vi "Read Batch Profiles(for High-Speed Mode).vi"(8 "error in (no error)":errorcluster, 9 "Data Size (0: Auto Size)":u32, 10 "Read Req":T2={"Read Area"=TRUE, "Batch Pos"=0, "Read Batch No"=0, "Read Profile No."=0, "Read Profile Cnt"=0, "Erase"=FALSE} {"Batch Pos" items=["CURRENT"=0, "SPECIFY"=2, "COMMITED"=3, "NEWEST PROFILE"=4]}, 11 "Device ID (0)":i32) -> (0 "error out":errorcluster, 1 "Profile Rsp":T1, 2 "Profile Data":u32[](array[numeric]), 3 "Device ID out":i32, 5 "Profile Info":T4={"Profile Cnt"=1, "Envelope"=FALSE, " Profile Data Point"=0, " X Start"=0, " X Pitch"=0})   [LabVIEW 2014, in "Keyence LJ-V7000.lvlib"]
doc: "This function gets profile data.\nProfile data is stored in 0.01 μm units.\n\n<B>Note</B>:\nFor the details on the data stored in the profile data (storage order and size), refer to <B>10.3</B> in a manual of measuring instrument drivers.\n\nIf Compression(timse axis) is ON, use <B>Read Profiles(for High-Speed Mode)</B> VI.\n\nTo read all of the profiles in one batch, read them with the procedure below.\n1. Call this VI by specifying <B>Current</B> for <B>Batch Pos</B> in <B>Read Req</B>. Save the start position and the amount of profiles that were read and the batch number that was read.\n2. Configure <B>Read Req</B> as listed below and call this VI again.\n　・<B>Batch Pos</B> = SPECIFY\n　・<B>Read Batch No</B> = batch number that was read\n　・<B>Read Profile Cnt</B> = starting profile number of the unread profiles in the batch\n3. Update <B>Read Profile Cnt</B> in step 2 and call this VI until all of the profiles in the batch can be read."
uses:
  Keyence LJ-V7000.lvlib
  Clusters/Profile Info.ctl
  Clusters/Read Batch Profile Req.ctl
  constant/Batch Pos.ctl
  Clusters/Read Batch Profile Rsp.ctl
  constant/Driver VI No.ctl
  Private/vi/Low Level/Make DLL Param(Read Batch Profile Req).vi
  Private/vi/Low Level/Make DLL Param(Read Batch Profile Rsp).vi
  Private/vi/Low Level/Make VI Param(Read Batch Profile Rsp).vi
panel:
  # "(c) 2012 KEYENCE CORPORATION.  ALL RIGHTS RESERVED."
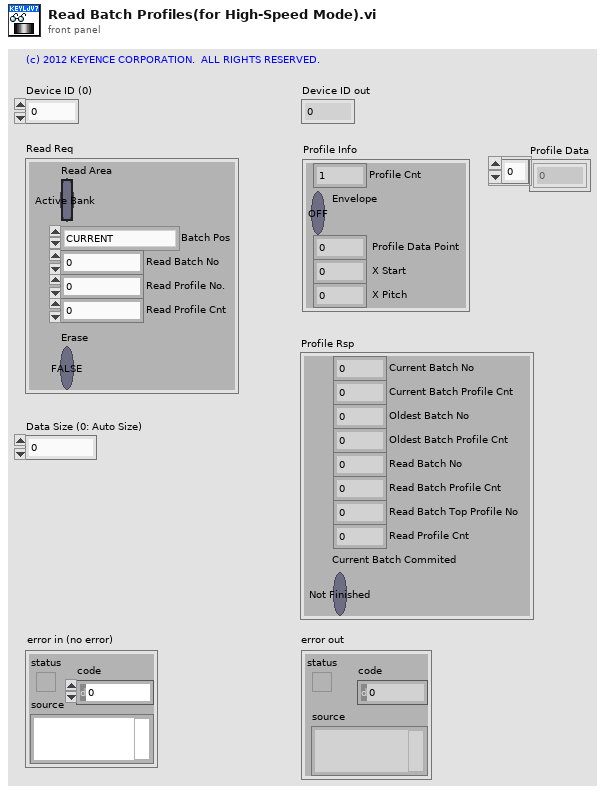
[diagram p1: front panel]
types:
  T1 = typedef "Keyence LJ-V7000.lvlib/Read Batch Profile Rsp.ctl" = cluster{"Current Batch No":u32, "Current Batch Profile Cnt":u32, "Oldest Batch No":u32, "Oldest Batch Profile Cnt":u32, "Read Batch No":u32, "Read Batch Profile Cnt":u32, "Read Batch Top Profile No":u32, "Read Profile Cnt":u8, "Current Batch Commited":bool}
  T2 = typedef "Keyence LJ-V7000.lvlib/Read Batch Profile Req.ctl" = cluster{"Read Area":bool, "Batch Pos":T3, "Read Batch No":u32, "Read Profile No.":u32, "Read Profile Cnt":u8, "Erase":bool}
  T3 = typedef "Keyence LJ-V7000.lvlib/Batch Pos.ctl" = u8
  T4 = typedef "Keyence LJ-V7000.lvlib/Profile Info.ctl" = cluster{"Profile Cnt":u8, "Envelope":bool, " Profile Data Point":u16, " X Start":i32, " X Pitch":i32}
  T5 = typedef "Keyence LJ-V7000.lvlib/Driver VI No.ctl" = enum16{"Initialize", "Close", "Reboot Controller", "Return to Factory State", "Get System Error", "Clear System Error", "Trigger", "Start Batch Measurements", "Stop Batch Measurements", "Auto Zero", "Timing", "Reset", "Clear Memory", "Set Setting", "Get Setting", "Initialize Setting", "Reflect Setting", "Update Write Settings Area", "Check Status of Saving to Save Area", "Set Time", "Get Time", "Change Program", "Read Active Program Number", "Read Measurement Data", "Read Profiles(for High-Speed Mode)", "Read Batch Profiles(for High-Speed Mode)", "Read Profiles(for Advanced Mode)", "Read Batch Profiles(for Advanced Mode)", "Start Storage", "Stop Storage", "Read Storage Status", "Read Data Storage Data", "Read Profile Storage Data", "Read Batch Profile Storage Data", "Start High-Speed Data Communication", "Stop High-Speed Data Communication", "Read Profiles(for High-Speed Communication)"}
  T6 = cluster{u8, "Batch Pos":T3, "reserve":u8, "reserve":u8, "Read Batch No":u32, "Read Profile No.":u32, "Read Profile Cnt":u8, u8, "reserve":u8, "reserve":u8}
  T7 = cluster{"Current Batch No":u32, "Current Batch Profile Cnt":u32, "Oldest Batch No":u32, "Oldest Batch Profile Cnt":u32, "Read Batch No":u32, "Read Batch Profile Cnt":u32, "Read Batch Top Profile No":u32, "Read Profile Cnt":u8, u8, "reserve":u8, "reserve":u8}
  T8 = cluster{"Profile Cnt":u8, u8, "reserve":u8, "reserve":u8, " Profile Data Point":u16, "reserve":u8, "reserve":u8, " X Start":i32, " XPitch":i32}
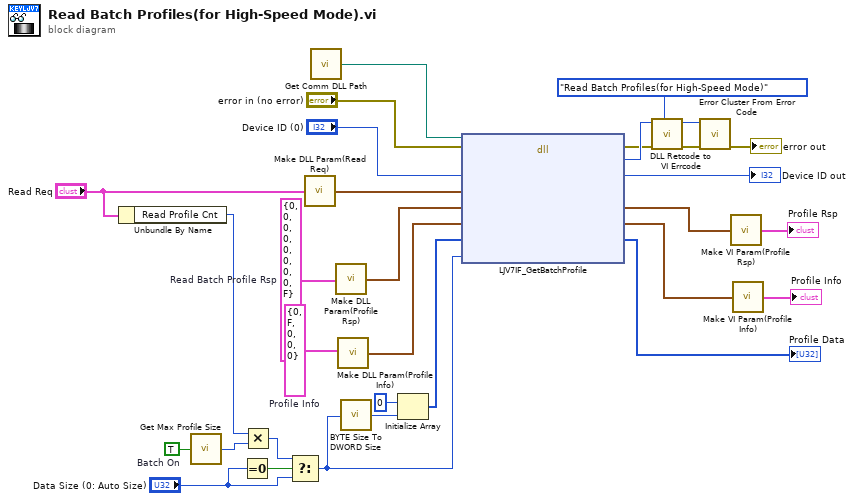
[diagram p0: block diagram]
diagram:
  w22 = T1 {"Current Batch No"=0, "Current Batch Profile Cnt"=0, "Oldest Batch No"=0, "Oldest Batch Profile Cnt"=0, "Read Batch No"=0, "Read Batch Profile Cnt"=0, "Read Batch Top Profile No"=0, "Read Profile Cnt"=0, "Current Batch Commited"=FALSE}  # Read Batch Profile Rsp
  w14 = TRUE  # Batch On
  w26 = T4 {"Profile Cnt"=0, "Envelope"=FALSE, " Profile Data Point"=0, " X Start"=0, " X Pitch"=0}  # Profile Info
  n1 = Unbundle By Name("Read Req") -> ("Read Profile Cnt"=w11:u8)
  n2 = call "Get Max Profile Size.vi"("Batch On-Off"=w14) -> ("Profile Size"=w13:u32)  [unwired: 4 in]
  n3 = Equal To 0?(x="Data Size (0: Auto Size)") -> (x = 0?=w16:bool)
  n4 = Multiply(x=w11, y=w13) -> (x*y=w10:u32)
  n5 = Select(t=w10, s=w16, f="Data Size (0: Auto Size)") -> (s? t:f=w7:u32)
  n6 = call-poly "Make DLL Param(Read Req).vi"("Read Batch Profile Req"="Read Req") -> ("pReq"=w24:T6)
  n7 = call "Get Comm DLL Path.vi"() -> ("Comm DLL Path"=w29:path)  [unwired: 1 in]
  n8 = call-poly "Make DLL Param(Profile Rsp).vi"("Read Batch Profile Rsp"=w22) -> ("pRsp"=w23:T7)
  n9 = call "Make DLL Param(Profile Info).vi"("Profile Info"=w26) -> ("DLL Parameter"=w25:T8)
  n10 = call "BYTE Size To DWORD Size.vi"("BYTE Size"=w7) -> ("DWORD Size"=w9:u32)
  n11 = Initialize Array(u32 0, w9) -> (w8:u32[])
  n12 = dll-call lib="C:/Program Files/National Instruments/LabVIEW 2011/instr.lib/Keyence LJ-V7000/LJV7_IF.*" fn="LJV7IF_GetBatchProfile"(path in=w29, error in="error in (no error)", "lDeviceId"="Device ID (0)", "pReq"=w24, "pRsp"=w23, "pProfileInfo"=w25, "pdwProfileData"=w8, "dwDataSize"=w7) -> (error out=w3:errorcluster, "lRetCode"=w4:i32, "lDeviceId"=→"Device ID out":i32, "pRsp"=w19:T7, "pProfileInfo"=w21:T8, "pdwProfileData"=→"Profile Data":u32[])  [unwired: 3 in, 1 out]
  n13 = call "DLL Retcode to VI Errcode.vi"("Driver VI No"=Driver_VI_No."Read Batch Profiles(for High-Speed Mode)", "error in (no error)"=w3, "DLL Return Code"=w4) -> ("error out"=w6:errorcluster, "VI Error Code"=w5:i32)  [unwired: 7 in]
  n14 = call <vilib>:"Error Cluster From Error Code.vi"("error in (no error)"=w6, "error code (0)"=w5) -> ("error out"=→"error out":errorcluster)  [unwired: 7 in]
  n15 = call-poly "Make VI Param(Profile Rsp).vi"("pRsp"=w19) -> ("Read Batch Profile Rsp"=→"Profile Rsp":T1)
  n16 = call "Make VI Param(Profile Info).vi"("pProfileInfo"=w21) -> ("Profile Info"=→"Profile Info":T4)
